vi "FPGA Main Image Processing - AXI.vi"(9 "?":T1) -> ()   [LabVIEW 2017]
doc: "The myRIO v1.1 FPGA Shipping Personality. This personality contains support for:\n- 2 Analog Input Interrupt channel\n- 4 Digital Input Interrupt channel\n- 1 Timer\n- 1 Accelerometer\n- 1 Button\n- 4 LED\n- 10 Analog Input channels with 1 Sample\n- 6 Analog Output channels with 1 Sample\n- 40 Digital I/O channels with 1 Sample\n- 2 I2C channels\n- 4 Encoder channels\n- 6 PWM channels\n- 2 SPI channels"
uses:
  <vilib>/rvi/DataTransferAndStorage/Container/XNode/niFpgaContainer.xnode
  <vilib>/rvi/LocalResourceManager/LocalResourceManager.xnode
  SoC IP Library/Controls/Image Size.ctl
  SoC IP Library/SoC IP Library.lvlib
  <vilib>/rvi/Memory/Memory_Emulation/nirvimemoryFastEmulation.vi
  <vilib>/rvi/Memory/Memory_Emulation/nirvimemoryEmulation.vi
  <vilib>/rvi/interface/RandomDataEmulation/nirviRandomDataFpgaReadWriteTemplate.vi
  <vilib>/rvi/DataTransferAndStorage/Container/Common/niFpgaContainerGetUniqueNameForEmu.vi
  <vilib>/rvi/DataTransferAndStorage/Container/Common/niFpgaContainerSetEmuInfo.vi
  <vilib>/rvi/eio/common/nirviEmuReportErrorAndStop.vi
  SoC IP Library/Controls/Ocurrences.ctl
panel:
  out "Write TO":bool
  out "Read TO":bool
  out "Pixel B Write":u32
  out "Pixel A Write":u32
  out "Last Processed Pixel?":bool
  out "Pixel":u32
  out "Processing iteration":i32=-1
  out "Current Colum Process":u32
  out "Current Row Process":u32
  out "Current Colum Write":u32
  out "Current Row Write":u32
  out "Last Write Pixel?":bool
  out "Last Read Pixel?":bool
  out "Current Colum Read":u32
  out "Current Row Read":u32
  out "Pixel B Write":u32
  out "Pixel A Write":u32
  out "Pixel B Read":u32
  out "Pixel A Read":u32
  out "SYS.OCURRENCES.RDY":bool
  out "FPGA to RT iteration":i32=-1
  out "RT to FPGA iteration":i32=-1
  out "SYS.IMG_SIZE.RDY":bool
  out "Image size":u32
  out "SYS.RDY":bool
  # "Image Processing"
  # "System"
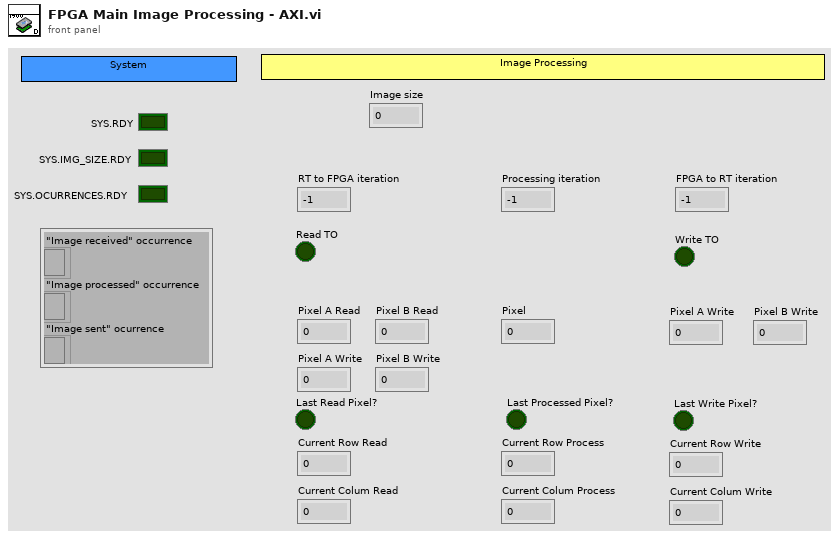
[diagram p1: front panel]
types:
  T1 = typedef "SoC IP Library.lvlib/Ocurrences.ctl" = cluster{"\"Image received\" occurrence":refnum<k4>, "\"Image processed\" occurrence":refnum<k4>, "\"Image sent\" ocurrence":refnum<k4>}
  T2 = typedef "SoC IP Library.lvlib/Image Size.ctl" = cluster{"Rows (X)":u16, "Colums (Y)":u16}
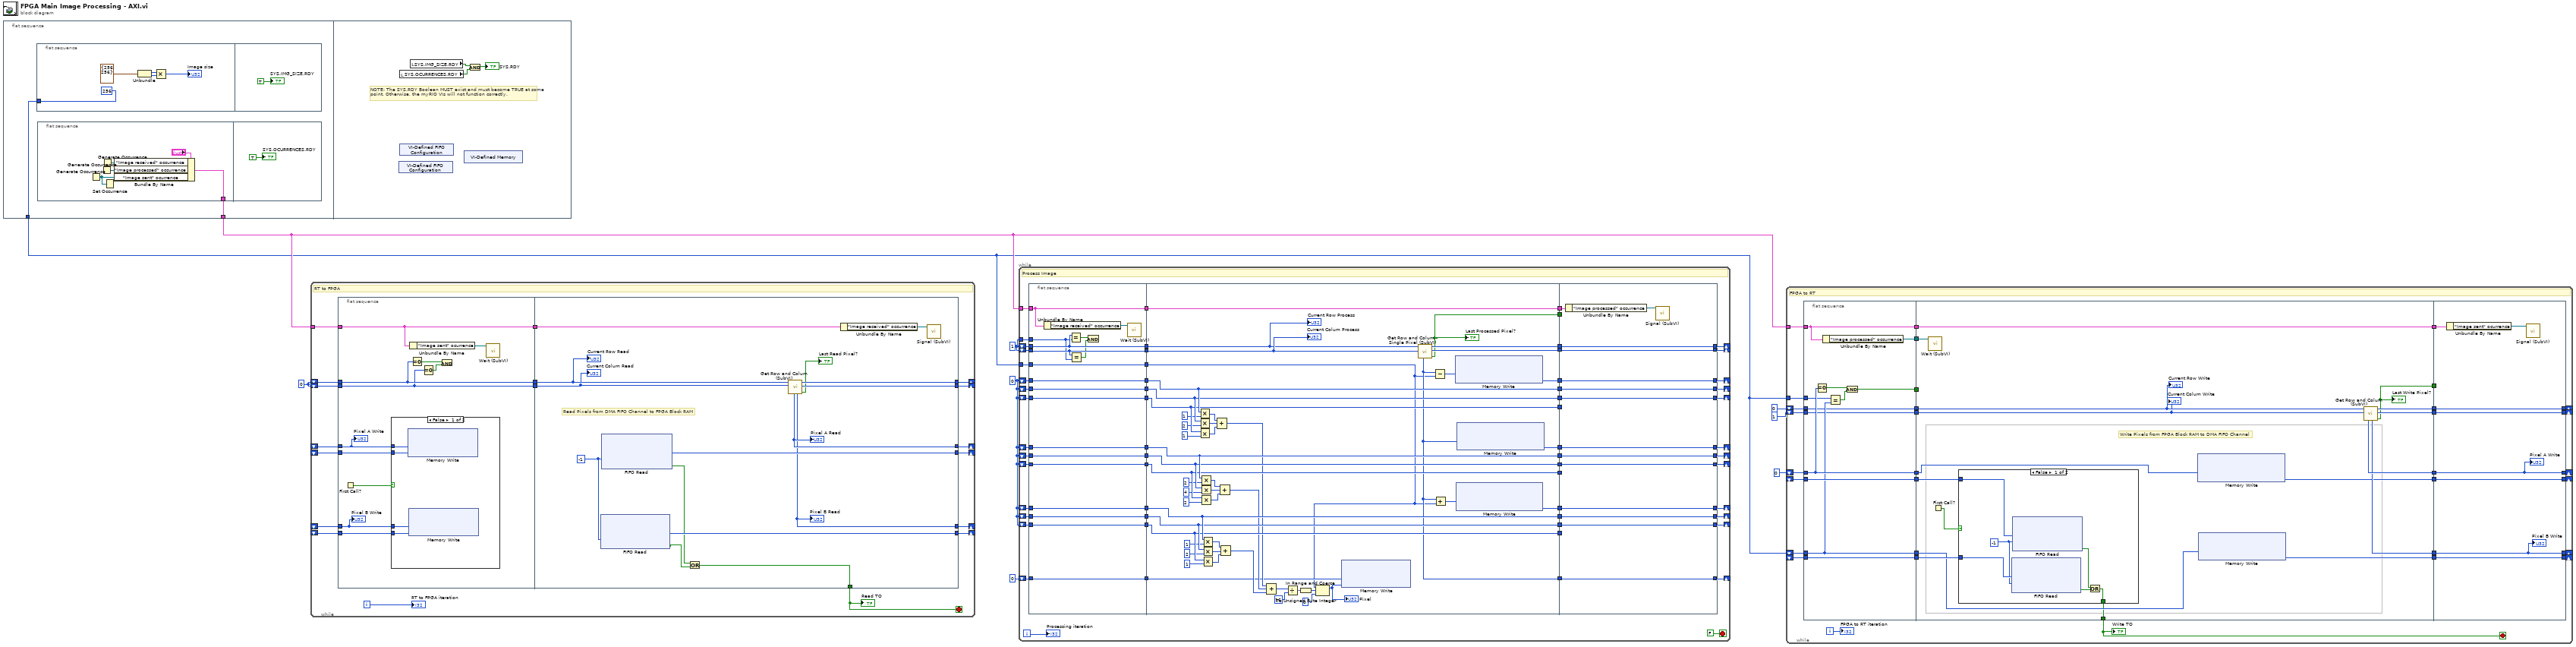
[diagram p0: block diagram]
diagram:
  w1 = u8 0 ("Data")
  w2 = u32 1 ("Row Out")
  w7 = u32 0
  n1 = flat-sequence {
    tunnel: [w11] -> w4
    tunnel: [w10] -> w5
    frame #0 {
      n2 = flat-sequence {
        tunnel: [u32 256 ("Dimension")] -> w11
        frame #0 {
          n3 = Unbundle(T2 {"Rows (X)"=256, "Colums (Y)"=256} ("Image Size")) -> ("Rows (X)"=w20:u16, "Colums (Y)"=w21:u16)
          n4 = Multiply(x=w20, y=w21) -> (x*y=→"Image size":u32)
        }
        frame #1 {
          "SYS.IMG_SIZE.RDY" <- TRUE
        }
      }
      n5 = flat-sequence {
        tunnel: [w12] -> w10
        frame #0 {
          n6 = Generate Occurrence() -> (w13:refnum<k4>)
          n7 = Generate Occurrence() -> (w14:refnum<k4>)
          n8 = Generate Occurrence() -> (w15:refnum<k4>)
          n9 = Set Occurrence(w13) -> ()
          n10 = Bundle By Name(cluster="?", "\"Image received\" occurrence"=w15, "\"Image processed\" occurrence"=w14, "\"Image sent\" ocurrence"=w13) -> (w12:T1)
        }
        frame #1 {
          "SYS.OCURRENCES.RDY" <- TRUE
        }
      }
    }
    frame #1 {
      # "NOTE: The SYS.RDY Boolean MUST exist and must become TRUE at some point. Otherwise, the myRIO VIs will not function correctly."
      n11 = xnode "VI-Defined FIFO Configuration"() -> ()  [unwired: 1 out]
      n12 = xnode "VI-Defined FIFO Configuration"() -> ()  [unwired: 1 out]
      n13 = local read "SYS.OCURRENCES.RDY"() -> (w25:bool)
      n14 = local read "SYS.IMG_SIZE.RDY"() -> (w24:bool)
      n15 = xnode "VI-Defined Memory"() -> ()  [unwired: 1 out]
      n16 = And(x=w24, y=w25) -> (x .and. y?=→"SYS.RDY":bool)
    }
  }
  n17 = while {
    shift-right: [w36] -> _
    shift-left: _ -> [w43]
    shift-right: [w30] -> _
    shift-left: _ -> [w42]
    shift-right: [w35] -> _
    shift-left: _ -> [w41]
    shift-right: [w39] -> _
    shift-left: _ -> [w40]
    shift-right: [w38] -> _
    shift-left: w7 -> [w34]
    shift-right: [w37] -> _
    shift-left: w7 -> [w33]
    tunnel: w5 -> [w29]
    i -> [w44]
    stop <- w27 stop-if-true
    # "RT to FPGA"
    n18 = flat-sequence {
      tunnel: w33 -> [w53]
      tunnel: w34 -> [w54]
      tunnel: w40 -> [w47]
      tunnel: w41 -> [w45]
      tunnel: w42 -> [w48]
      tunnel: w43 -> [w46]
      tunnel: [w54] -> w32
      tunnel: [w53] -> w31
      tunnel: w29 -> [w55]
      tunnel: [w55] -> w28
      tunnel: w32 -> [w70]
      tunnel: w31 -> [w69]
      tunnel: w28 -> [w67]
      tunnel: [w74] -> w30
      tunnel: [w73] -> w39
      tunnel: [w72] -> w38
      tunnel: [w71] -> w37
      tunnel: [w66] -> w36
      tunnel: [w65] -> w35
      tunnel: [w61] -> w27
      frame #0 {
        n19 = First Call?() -> (First Call?: T/F=w49:bool)
        n20 = case shown="False" w49 {
          tunnel: w46 -> [w59 _]
          tunnel: w48 -> [w57 _]
          tunnel: w47 -> [w56 _]
          tunnel: w45 -> [w58 _]
          frame False {
            n21 = xnode ("Memory Write")("Address"=w59, "Data"=w57) -> ()  [unwired: 1 in, 1 out]
            n22 = xnode ("Memory Write")("Address"=w58, "Data"=w56) -> ()  [unwired: 1 in, 1 out]
          }
          frame True {
          }
        }
        n23 = Unbundle By Name(w55) -> ("\"Image sent\" ocurrence"=w51:refnum<k4>)
        n24 = Equal To 0?(x=w54) -> (x = 0?=w52:bool)
        n25 = Equal To 0?(x=w53) -> (x = 0?=w50:bool)
        n26 = And(x=w52, y=w50) -> ()  [unwired: 1 out]
        n27 = call "Wait (SubVI).vi"("Occurrence in"=w51) -> ()  [unwired: 11 in]
        "Pixel A Write" <- w46
        "Pixel B Write" <- w45
      }
      frame #1 {
        w60 = -1 ("Timeout")
        # "Read Pixels from DMA FIFO Channel to FPGA Block RAM"
        n28 = xnode ("FIFO Read")("Timeout"=w60) -> ("Element"=w73:u8, "Timed Out?"=w62:bool)  [unwired: 1 in, 1 out]
        n29 = xnode ("FIFO Read")("Timeout"=w60) -> ("Element"=w74:u8, "Timed Out?"=w63:bool)  [unwired: 1 in, 1 out]
        n30 = Or(x=w63, y=w62) -> (x .or. y?=w61:bool)
        n31 = call "Get Row and Colum (SubVI).vi"("Colum In"=w69, "Row In"=w70) -> ("Last Pixel?"=→"Last Read Pixel?":bool, "Colum Out"=w71:u8, "Row Out"=w72:u8, "Pixel B"=w65:u16, "Pixel A"=w66:u16)  [unwired: 5 in]
        "Pixel A Read" <- w66
        "Pixel B Read" <- w65
        n32 = Unbundle By Name(w67) -> ("\"Image received\" occurrence"=w64:refnum<k4>)
        n33 = call "Signal (SubVI).vi"("Occurrence in"=w64) -> ()  [unwired: 11 in]
        "Current Row Read" <- w70
        "Current Colum Read" <- w69
      }
    }
    "RT to FPGA iteration" <- w44
    "Read TO" <- w27
  }
  n34 = while {
    tunnel: w5 -> [w133]
    shift-right: [w129] -> _
    shift-left: w1 -> [w127]
    shift-right: [w125] -> _
    shift-left: w1 -> [w124]
    shift-right: [w121] -> _
    shift-left: w1 -> [w119]
    shift-right: [w116] -> _
    shift-left: w1 -> [w114]
    shift-right: [w112] -> _
    shift-left: w1 -> [w110]
    shift-right: [w108] -> _
    shift-left: w1 -> [w106]
    shift-right: [w103] -> _
    shift-left: w1 -> [w102]
    shift-right: [w99] -> _
    shift-left: w1 -> [w98]
    shift-right: [w95] -> _
    shift-left: w1 -> [w93]
    shift-right: [w90] -> _
    shift-left: w2 -> [w85]
    shift-right: [w88] -> _
    shift-left: w2 -> [w86]
    tunnel: w4 -> [w83]
    shift-right: [w79] -> _
    shift-left: u32 0 ("Pixel") -> [w81]
    tunnel: w2 -> [w77]
    i -> [w75]
    stop <- FALSE stop-if-true
    # "Process Image"
    n35 = flat-sequence {
      tunnel: w133 -> [w151]
      tunnel: [w151] -> w131
      tunnel: [w150] -> w128
      tunnel: w127 -> [w150]
      tunnel: w124 -> [w149]
      tunnel: [w149] -> w123
      tunnel: [w148] -> w120
      tunnel: w119 -> [w148]
      tunnel: [w147] -> w115
      tunnel: w114 -> [w147]
      tunnel: [w146] -> w111
      tunnel: w110 -> [w146]
      tunnel: [w145] -> w107
      tunnel: w106 -> [w145]
      tunnel: w102 -> [w144]
      tunnel: [w144] -> w101
      tunnel: w98 -> [w143]
      tunnel: [w143] -> w97
      tunnel: [w142] -> w94
      tunnel: w93 -> [w142]
      tunnel: [w139] -> w87
      tunnel: w86 -> [w139]
      tunnel: w85 -> [w138]
      tunnel: [w138] -> w84
      tunnel: w83 -> [w141]
      tunnel: [w141] -> w82
      tunnel: w81 -> [w140]
      tunnel: [w140] -> w80
      tunnel: w77 -> [w137]
      tunnel: [w202] -> w132
      tunnel: w131 -> [w202]
      tunnel: [w201] -> w130
      tunnel: w128 -> [w198]
      tunnel: [w198] -> w126
      tunnel: w123 -> [w197]
      tunnel: [w197] -> w122
      tunnel: w120 -> [w196]
      tunnel: [w196] -> w118
      tunnel: [w200] -> w117
      tunnel: w115 -> [w195]
      tunnel: [w195] -> w113
      tunnel: w111 -> [w194]
      tunnel: [w194] -> w109
      tunnel: w107 -> [w193]
      tunnel: [w193] -> w105
      tunnel: [w199] -> w104
      tunnel: w101 -> [w192]
      tunnel: [w192] -> w100
      tunnel: w97 -> [w191]
      tunnel: [w191] -> w96
      tunnel: w94 -> [w190]
      tunnel: [w190] -> w92
      tunnel: [w168] -> w91
      tunnel: [w167] -> w89
      tunnel: w87 -> [w158]
      tunnel: w84 -> [w159]
      tunnel: w82 -> [w160]
      tunnel: w80 -> [w164]
      tunnel: [w163] -> w78
      tunnel: [w157] -> w76
      tunnel: w132 -> [w216]
      tunnel: w130 -> [w214]
      tunnel: [w214] -> w129
      tunnel: w126 -> [w213]
      tunnel: [w213] -> w125
      tunnel: w122 -> [w212]
      tunnel: [w212] -> w121
      tunnel: w118 -> [_]
      tunnel: w117 -> [w211]
      tunnel: [w211] -> w116
      tunnel: w113 -> [w210]
      tunnel: [w210] -> w112
      tunnel: w109 -> [w209]
      tunnel: [w209] -> w108
      tunnel: w105 -> [_]
      tunnel: w104 -> [w208]
      tunnel: [w208] -> w103
      tunnel: w100 -> [w207]
      tunnel: [w207] -> w99
      tunnel: w96 -> [w206]
      tunnel: [w206] -> w95
      tunnel: w92 -> [_]
      tunnel: [w205] -> w90
      tunnel: w91 -> [w205]
      tunnel: w89 -> [w204]
      tunnel: [w204] -> w88
      tunnel: [w203] -> w79
      tunnel: w78 -> [w203]
      tunnel: w76 -> [_]
      frame #0 {
        n36 = Unbundle By Name(w151) -> ("\"Image received\" occurrence"=w152:refnum<k4>)
        n37 = Equal?(x=w139, y=w137) -> (x = y?=w136:bool)
        n38 = Equal?(x=w138, y=w137) -> (x = y?=w135:bool)
        n39 = And(x=w136, y=w135) -> ()  [unwired: 1 out]
        n40 = call "Wait (SubVI).vi"("Occurrence in"=w152) -> ()  [unwired: 11 in]
      }
      frame #1 {
        n41 = Multiply(x=w198, y=i16 1) -> (x*y=w184:i16)
        n42 = Multiply(x=w197, y=i16 2) -> (x*y=w186:i16)
        n43 = Multiply(x=w196, y=i16 1) -> (x*y=w185:i16)
        n44 = Multiply(x=w195, y=i16 2) -> (x*y=w183:i16)
        n45 = Multiply(x=w194, y=i16 4) -> (x*y=w182:i16)
        n46 = Multiply(x=w193, y=i16 2) -> (x*y=w181:i16)
        n47 = Multiply(x=w192, y=i16 1) -> (x*y=w189:i16)
        n48 = Multiply(x=w191, y=i16 2) -> (x*y=w188:i16)
        n49 = Multiply(x=w190, y=i16 1) -> (x*y=w187:i16)
        n50 = Compound Arithmetic op=ADD(w184, w186, w185) -> (w180:i16)
        n51 = Compound Arithmetic op=ADD(w183, w182, w181) -> (w179:i16)
        n52 = Compound Arithmetic op=ADD(w189, w188, w187) -> (w178:i16)
        n53 = Compound Arithmetic op=ADD(w180, w179, w178) -> (w156:i16)
        n54 = Divide(x=w156, y=i16 16) -> (x/y=w154:fxp<+,8,8>)
        n55 = To Unsigned Byte Integer(number=w154) -> (unsigned 8bit integer=w153:u8)
        n56 = In Range and Coerce(upper limit=w160, x=w153, lower limit=i16 0) -> (coerced(x)=w162:u32)  [unwired: 1 out]
        "Pixel" <- w162
        n57 = xnode ("Memory Write")("Address"=w164, "Data"=w162) -> ()  [unwired: 1 in, 1 out]
        n58 = call "Get Row and Colum - Single Pixel (SubVI).vi"("Colum In"=w159, "Row In"=w158) -> ("Last Pixel?"=w157:bool, "Colum Out"=w168:u8, "Row Out"=w167:u8, "Pixel"=w163:u16)  [unwired: 6 in]
        "Last Processed Pixel?" <- w157
        n59 = Subtract(x=w163, y=w160) -> (x-y=w165:u32)
        n60 = Add(x=w163, y=w160) -> (x+y=w166:u32)
        n61 = xnode ("Memory Write")("Address"=w165) -> ("Data"=w201:u8)  [unwired: 1 in, 1 out]
        n62 = xnode ("Memory Write")("Address"=w166) -> ("Data"=w199:u8)  [unwired: 1 in, 1 out]
        n63 = xnode ("Memory Write")("Address"=w163) -> ("Data"=w200:u8)  [unwired: 1 in, 1 out]
        "Current Row Process" <- w158
        "Current Colum Process" <- w159
      }
      frame #2 {
        n64 = Unbundle By Name(w216) -> ("\"Image processed\" occurrence"=w215:refnum<k4>)
        n65 = call "Signal (SubVI).vi"("Occurrence in"=w215) -> ()  [unwired: 11 in]
      }
    }
    "Processing iteration" <- w75
  }
  n66 = while {
    shift-right: [w245] -> _
    shift-left: u32 0 -> [w249]
    shift-right: [w244] -> _
    shift-left: w4 -> [w248]
    shift-right: [w247] -> _
    shift-left: u32 0 -> [w243]
    shift-right: [w246] -> _
    shift-left: u32 1 ("Colum Out") -> [w242]
    shift-right: [w232] -> _
    shift-left: _ -> [w228]
    shift-right: [w230] -> _
    shift-left: _ -> [w226]
    tunnel: w4 -> [w222]
    tunnel: w5 -> [w221]
    i -> [w234]
    stop <- w217 stop-if-true
    # "FPGA to RT"
    n67 = flat-sequence {
      tunnel: w242 -> [w253]
      tunnel: w243 -> [w254]
      tunnel: w248 -> [w256]
      tunnel: w249 -> [w257]
      tunnel: [w257] -> w241
      tunnel: [w256] -> w240
      tunnel: [w259] -> w229
      tunnel: w228 -> [w259]
      tunnel: [w258] -> w227
      tunnel: w226 -> [w258]
      tunnel: [w255] -> w225
      tunnel: [w254] -> w224
      tunnel: [w253] -> w223
      tunnel: w222 -> [w252]
      tunnel: w221 -> [w251]
      tunnel: [w251] -> w220
      tunnel: [w250] -> w218
      tunnel: w241 -> [w268]
      tunnel: w240 -> [w267]
      tunnel: [w278] -> w239
      tunnel: [w277] -> w238
      tunnel: [w276] -> w237
      tunnel: [w275] -> w236
      tunnel: [w274] -> w235
      tunnel: [w273] -> w233
      tunnel: [w272] -> w231
      tunnel: w229 -> [w271]
      tunnel: w227 -> [w270]
      tunnel: w225 -> [_]
      tunnel: w224 -> [w266]
      tunnel: w223 -> [w265]
      tunnel: w220 -> [w264]
      tunnel: [w264] -> w219
      tunnel: w218 -> [w263]
      tunnel: [w262] -> w217
      tunnel: [w289] -> w244
      tunnel: [w290] -> w245
      tunnel: [w291] -> w246
      tunnel: [w292] -> w247
      tunnel: w239 -> [w292]
      tunnel: w238 -> [w291]
      tunnel: w237 -> [w290]
      tunnel: w236 -> [w289]
      tunnel: w235 -> [_]
      tunnel: [w288] -> w232
      tunnel: w233 -> [w288]
      tunnel: [w287] -> w230
      tunnel: w231 -> [w287]
      tunnel: w219 -> [w286]
      frame #0 {
        n68 = Equal To 0?(x=w257) -> (x = 0?=w260:bool)
        n69 = Unbundle By Name(w251) -> ("\"Image processed\" occurrence"=w250:refnum<k4>)
        n70 = Equal?(x=w252, y=w256) -> (x = y?=w261:bool)
        n71 = And(x=w260, y=w261) -> (x .and. y?=w255:bool)
      }
      frame #1 {
        # "Write Pixels from FPGA Block RAM to DMA FIFO Channel"
        n72 = call "Wait (SubVI).vi"("Occurrence in"=w263) -> ()  [unwired: 11 in]
        n73 = First Call?() -> (First Call?: T/F=w269:bool)
        n74 = case shown="False" w269 {
          tunnel: w271 -> [w284 _]
          tunnel: w270 -> [w283 _]
          tunnel: [w280 _] -> w262
          frame False {
            w279 = -1 ("Timeout")
            n75 = xnode ("FIFO Read")("Element"=w283, "Timeout"=w279) -> ("Timed Out?"=w282:bool)  [unwired: 1 in, 1 out]
            n76 = xnode ("FIFO Read")("Element"=w284, "Timeout"=w279) -> ("Timed Out?"=w281:bool)  [unwired: 1 in, 1 out]
            n77 = Or(x=w281, y=w282) -> (x .or. y?=w280:bool)
          }
          frame True {
          }
        }
        n78 = xnode ("Memory Write")("Address"=w268) -> ("Data"=w273:u8)  [unwired: 1 in, 1 out]
        n79 = xnode ("Memory Write")("Address"=w267) -> ("Data"=w272:u8)  [unwired: 1 in, 1 out]
        n80 = call "Get Row and Colum (SubVI).vi"("Colum In"=w265, "Row In"=w266) -> ("Last Pixel?"=w274:bool, "Colum Out"=w277:u8, "Row Out"=w278:u8, "Pixel B"=w275:u16, "Pixel A"=w276:u16)  [unwired: 5 in]
        "Last Write Pixel?" <- w274
        "Current Row Write" <- w266
        "Current Colum Write" <- w265
      }
      frame #2 {
        n81 = Unbundle By Name(w286) -> ("\"Image sent\" ocurrence"=w285:refnum<k4>)
        n82 = call "Signal (SubVI).vi"("Occurrence in"=w285) -> ()  [unwired: 11 in]
        "Pixel A Write" <- w290
        "Pixel B Write" <- w289
      }
    }
    "FPGA to RT iteration" <- w234
    "Write TO" <- w217
  }
